vi "testresume.vi"   [LabVIEW 2011]
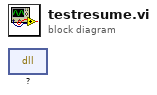
[diagram p0: block diagram]
diagram:
  n1 = dll-call lib="?" fn="?"() -> ()  [unwired: 4 in, 2 out]
